vi "myRIO_BRig_RT_dataTrial_CueLed.vi"() -> (2 "output_CueLed":i32)   [LabVIEW 2014]
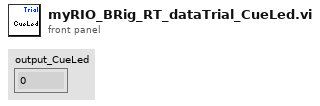
[diagram p1: front panel]
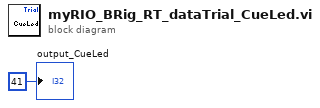
[diagram p0: block diagram]
diagram:
  "output_CueLed" <- 41 ("output_iBlock")
